vi "7HP_Channels.vi"(0 "Analysis Info cluster":T3[](array[typedef]) {"Sync Delay Time (s)" format="%.4f"; "Sd Error in Variance" format="%.2f"; "Skew_u" format="%.2f"; "% u'/U" format="%.2f"; "Sd Error in Mean" format="%.2f"; "Kurt_u" format="%.2f"; "u^4" format="%.2f"; "u^3" format="%.2f"; "U" format="%.2f"; "u^2" format="%.2f"}) -> (1 "Device port info":T1[](array[typedef]), 2 "7HP Info":T2(array[cluster]))   [LabVIEW 2018]
uses:
  Controls/Analysis_info_cluster.ctl
  Controls/Inst_type.ctl
  Controls/Instrument_Array.ctl
  Device ID port info.ctl
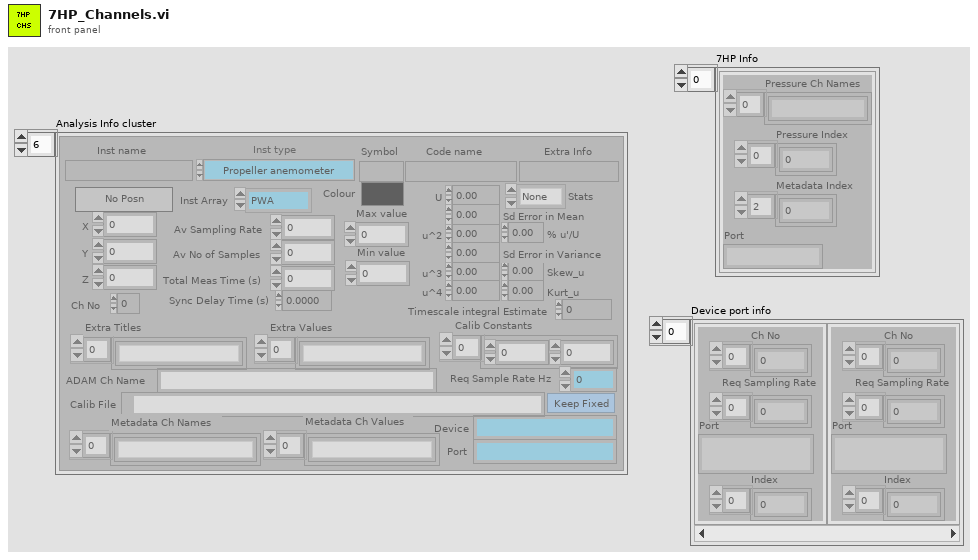
[diagram p1: front panel]
types:
  T1 = typedef "Device ID port info.ctl" = cluster{"Ch No":i16[], "Req Sampling Rate":dbl[], "Port":string, "Index":i32[]}
  T2 = cluster{"Pressure Ch Names":string[], "Pressure Index":i32[], "Metadata Index":i32[], "Port":string}[]
  T3 = typedef "Analysis_info_cluster.ctl" = cluster{"Colour":u32, "Inst type":T4, "Inst name":string, "Symbol":string, "Code name":string, "Extra Info":string, "Inst Array":T5, "Extra Titles":string[], "Extra Values":string[], "U":dbl, "u^2":dbl, "u^3":dbl, "u^4":dbl, "Skew_u":dbl, "Kurt_u":dbl, "Sd Error in Mean":dbl, "% u'/U":dbl, "X":dbl, "Y":dbl, "Z":dbl, "Timescale integral Estimate":dbl, "Sd Error in Variance":dbl, "Calib File":path, "Calib Constants":dbl[], "Output Position":bool, "Stats":enum16{"None", "Basic", "Full"}, "Av Sampling Rate":dbl, "Av No of Samples":dbl, "Total Meas Time (s)":dbl, "ADAM Ch Name":string, "Max value":dbl, "Min value":dbl, "Req Sample Rate Hz":dbl, "Sync Delay Time (s)":dbl, "Ch No":i16, "Device":string, "Use Latest Calib":bool, "Port":string, "Metadata Ch Names":string[], "Metadata Ch Values":string[]}
  T4 = typedef "Inst_type.ctl" = enum16{"Propeller anemometer", "Raw voltage", "Pressure Transducer", "Pitot-static tube", "Preston tube", "Hot wire", "Cross wire 1", "Cross wire 2", "Generic Linear", "Generic Polynomial", "Generic BackPoly", "Fast FID", "Thermocouple", "Cold wire", "Pulsed Wire", "LDA Vel", "LDA Tran time", "LDA Arr time", "Microphone"}
  T5 = typedef "Instrument_Array.ctl" = enum16{"PWA", "LDA", "Analogue"}
  T6 = cluster{"Pressure Ch Names":string[], "Pressure Index":i32[], "Metadata Index":i32[], "Port":string}
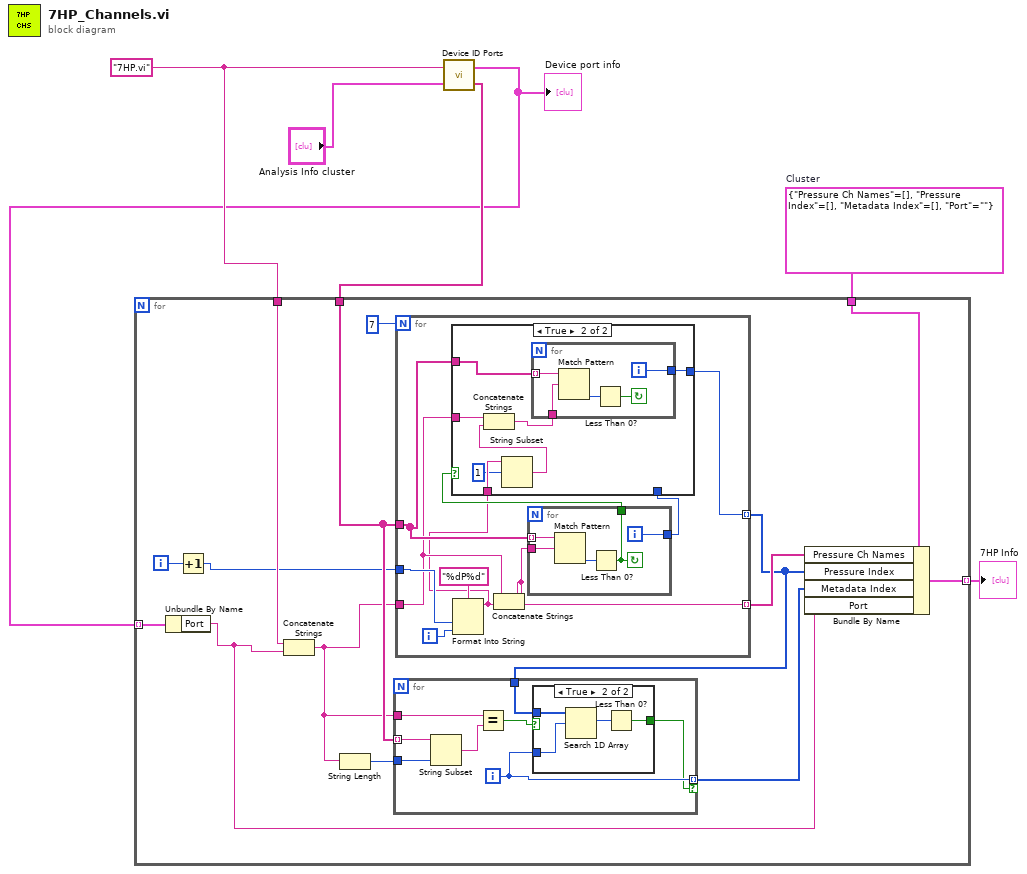
[diagram p0: block diagram]
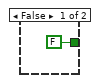
[diagram p2: hidden frame]
diagram:
  w3 = T6 {"Pressure Ch Names"=[], "Pressure Index"=[], "Metadata Index"=[], "Port"=""}  # Cluster
  w5 = "7HP.vi" ("Device ID")
  n1 = call "Device ID Ports.vi"("Analysis Info cluster"="Analysis Info cluster", "Device ID"=w5) -> ("Unique Channel Names"=w4:string[], "Device port info"=w1:T1[])
  "Device port info" <- w1
  n2 = for {
    tunnel: w5 -> [w20]
    tunnel: w4 -> [w15]
    tunnel: w3 -> [w18]
    tunnel: [w11] -> w2 mode=indexing
    tunnel: w1 -> [w10] mode=indexing
    i -> [w8]
    n3 = Unbundle By Name(w10) -> ("Port"=w9:string)
    n4 = Increment(x=w8) -> (x+1=w7:i32)
    n5 = Concatenate Strings(w20, w9) -> (w14:string)
    n6 = String Length(string=w14) -> (length=w16:i32)
    n7 = for {
      N: 7 -> [_]
      tunnel: w15 -> [w39]
      tunnel: [w38] -> w13 mode=indexing
      tunnel: w14 -> [w36]
      tunnel: [w35] -> w17 mode=indexing
      tunnel: w7 -> [w42]
      i -> [w41]
      n8 = Format Into String(format string="%dP%d", w42, w41) -> (resulting string=w34:string)  [unwired: 2 in, 1 out]
      n9 = Concatenate Strings(w36, w34) -> (w35:string)
      n10 = for {
        tunnel: w39 -> [w58] mode=indexing
        tunnel: w35 -> [w61]
        tunnel: [w59] -> w37
        tunnel: [w57] -> w40
        i -> [w59]
        stop <- w57 continue-if-true
        n11 = Match Pattern(string=w58, regular expression=w61) -> (offset past match=w60:i32)  [unwired: 1 in, 3 out]
        n12 = Less Than 0?(x=w60) -> (x < 0?=w57:bool)
      }
      n13 = case shown="True" w40 {
        tunnel: w39 -> [_ w51]
        tunnel: w34 -> [_ w50]
        tunnel: [w44 w48] -> w38
        tunnel: w37 -> [w44 _]
        tunnel: w36 -> [_ w46]
        frame False {
        }
        frame True {
          n14 = String Subset(string=w50, offset (0)=1) -> (substring=w47:string)  [unwired: 1 in]
          n15 = Concatenate Strings(w46, w47) -> (w45:string)
          n16 = for {
            tunnel: [w55] -> w48
            tunnel: w51 -> [w53] mode=indexing
            tunnel: w45 -> [w52]
            i -> [w55]
            stop <- w54 continue-if-true
            n17 = Match Pattern(string=w53, regular expression=w52) -> (offset past match=w56:i32)  [unwired: 1 in, 3 out]
            n18 = Less Than 0?(x=w56) -> (x < 0?=w54:bool)
          }
        }
      }
    }
    n19 = for {
      tunnel: w16 -> [w28]
      tunnel: w15 -> [w27] mode=indexing
      tunnel: w14 -> [w25]
      tunnel: w13 -> [w23]
      tunnel: [w22] -> w12 mode=indexing if=w21
      i -> [w22]
      n20 = String Subset(string=w27, length (rest)=w28) -> (substring=w26:string)  [unwired: 1 in]
      n21 = Equal?(x=w25, y=w26) -> (x = y?=w24:bool)
      n22 = case shown="True" w24 {
        tunnel: w23 -> [_ w33]
        tunnel: w22 -> [_ w32]
        tunnel: [FALSE w30] -> w21
        frame False {
        }
        frame True {
          n23 = Search 1D Array(1D array=w33, element=w32) -> (index of element=w31:i32)  [unwired: 1 in]
          n24 = Less Than 0?(x=w31) -> (x < 0?=w30:bool)
        }
      }
    }
    n25 = Bundle By Name(cluster=w18, "Pressure Ch Names"=w17, "Pressure Index"=w13, "Metadata Index"=w12, "Port"=w9) -> (w11:T6)
  }
  "7HP Info" <- w2
